vi "GetODBData.vi"(8 "error in (no error)":errorcluster, 11 "input cluster":T1) -> (0 "error out":errorcluster, 3 "MIDAS_ODB_Entry":T1)   [LabVIEW 2018, in "feGEM DataPacker.lvlib"]
uses:
  feGEM DataPacker.lvlib
  DataPacker/DataStructures/MIDAS_ODB_Entry.ctl
  DataPacker/GlobalVariables/MIDAS_ODB_Set_Get_Clear_Enum.ctl
panel:
  in  "Timeout after n trys (default = 100 (10s))":i32=100
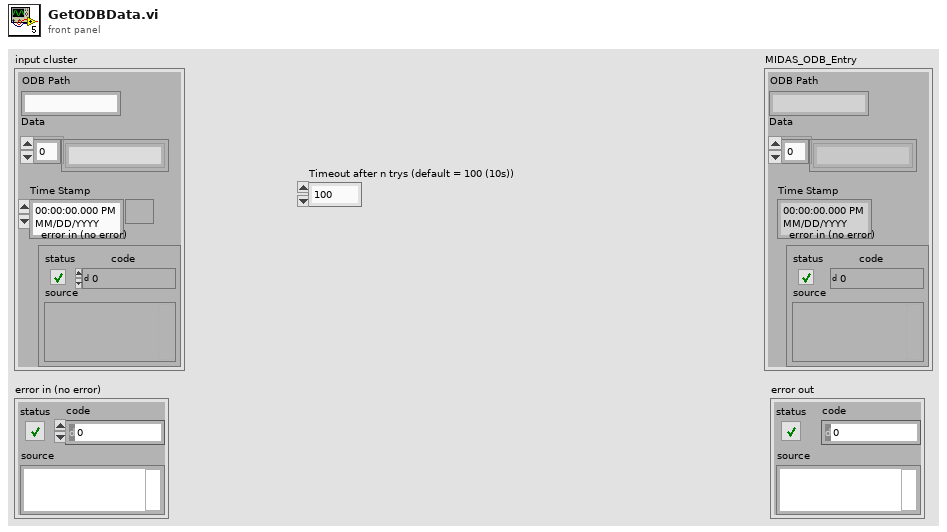
[diagram p1: front panel]
types:
  T1 = typedef "feGEM DataPacker.lvlib/MIDAS_ODB_Entry.ctl" = cluster{"ODB Path":string, "Data":string[], "Time Stamp":timestamp, "error in (no error)":errorcluster}
  T2 = typedef "feGEM DataPacker.lvlib/MIDAS_ODB_Set_Get_Clear_Enum.ctl" = enum16{"Set", "Get", "Clear"}
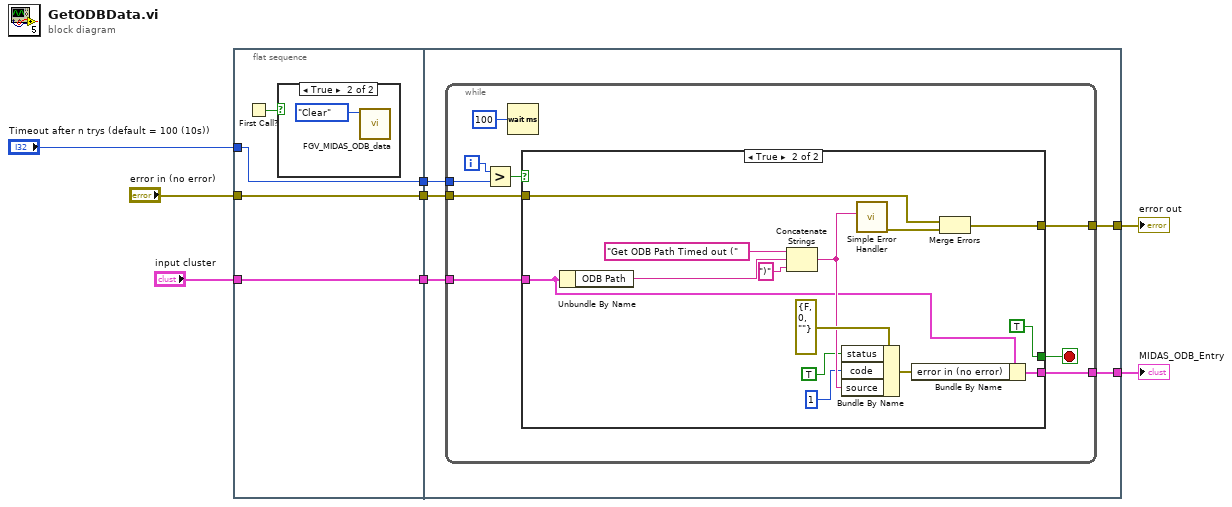
[diagram p0: block diagram]
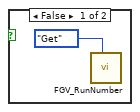
[diagram p2: hidden frame]
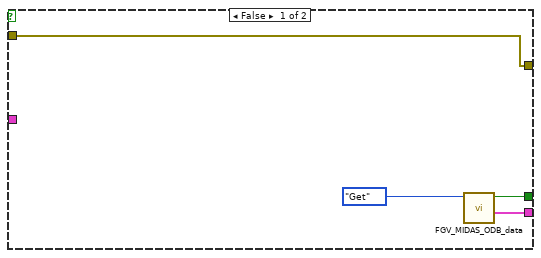
[diagram p3: hidden frame]
diagram:
  n1 = flat-sequence {
    tunnel: "Timeout after n trys (default = 100 (10s))" -> [w11]
    tunnel: [w11] -> w6
    tunnel: [w10] -> w5
    tunnel: "error in (no error)" -> [w10]
    tunnel: [w9] -> w3
    tunnel: "input cluster" -> [w9]
    tunnel: [w19] -> w8
    tunnel: [w18] -> w7
    tunnel: w6 -> [w17]
    tunnel: w5 -> [w16]
    tunnel: w3 -> [w15]
    frame #0 {
      n2 = First Call?() -> (First Call?: T/F=w12:bool)
      n3 = case shown="True" w12 {
        frame False {
          n4 = call "FGV_RunNumber.vi"("Enum"=enum16{"Set", "Get"}."Get") -> ()  [unwired: 4 in, 1 out]
        }
        frame True {
          n5 = call "FGV_MIDAS_ODB_data.vi"("Enum"=MIDAS_ODB_Set_Get_Clear_Enum."Clear") -> ()  [unwired: 9 in, 2 out]
        }
      }
    }
    frame #1 {
      n6 = while {
        tunnel: w16 -> [w25]
        tunnel: [w24] -> w19
        tunnel: w17 -> [w23]
        tunnel: [w21] -> w18
        tunnel: w15 -> [w22]
        i -> [w27]
        stop <- w20 stop-if-true
        n7 = Greater?(x=w27, y=w23) -> (0:w26:bool)
        n8 = Wait (ms)(milliseconds to wait=u32 100) -> ()  [unwired: 1 out]
        n9 = case shown="True" w26 {
          tunnel: w25 -> [w32 w46]
          tunnel: [w32 w44] -> w24
          tunnel: w22 -> [_ w36]
          tunnel: [w31 w33] -> w21
          tunnel: [w30 TRUE] -> w20
          frame False {
            n10 = call "FGV_MIDAS_ODB_data.vi"("Enum"=MIDAS_ODB_Set_Get_Clear_Enum."Get") -> ("MIDAS_ODB_Entry"=w31:T1, "Found Entry"=w30:bool)  [unwired: 9 in]
          }
          frame True {
            n11 = Unbundle By Name(w36) -> ("ODB Path"=w42:string)
            n12 = Concatenate Strings("Get ODB Path Timed out (" ("error source (\" \")"), w42, ")" ("string")) -> (w39:string)
            n13 = Bundle By Name(cluster=errorcluster {"status"=FALSE, "code"=0, "source"=""} ("error out"), "status"=TRUE, "code"=1, "source"=w39) -> (w35:errorcluster)
            n14 = call <vilib>:"Simple Error Handler.vi"("error source (\" \")"=w39) -> ("error out"=w45:errorcluster)  [unwired: 4 in, 4 out]
            n15 = Bundle By Name(cluster=w36, "error in (no error)"=w35) -> (w33:T1)
            n16 = Merge Errors(w46, w45) -> (w44:errorcluster)
          }
        }
      }
    }
  }
  "error out" <- w8
  "MIDAS_ODB_Entry" <- w7
